vi "tsdiag_set_stmin.vi"(8 "error in (no error)":errorcluster, 9 "AST":i32, 10 "ADiagModuleIndex":i32, 11 "路径输入":path) -> (0 "error out":errorcluster, 2 "retirn":i32, 3 "路径输出":path)   [LabVIEW 2014]
panel:
  # "e"
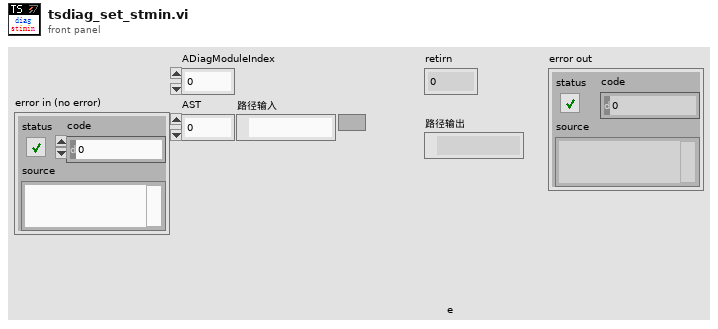
[diagram p1: front panel]
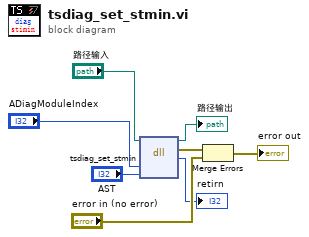
[diagram p0: block diagram]
diagram:
  n1 = dll-call lib="D:/Program Files (x86)/TOSUN/TSMaster/bin/TSMaster.dll" fn="tsdiag_set_stmin"(path in="路径输入", "ADiagModuleIndex"="ADiagModuleIndex", "AST"="AST") -> (path out=→"路径输出":path, error out=w8:errorcluster, "ACode"=→"retirn":i32)  [unwired: 4 in]
  n2 = Merge Errors(w8, "error in (no error)") -> (→"error out":errorcluster)
